vi "Temperature Warnings_EX.vi"() -> ()   [LabVIEW 2021]
doc: "This VI is used to determine the string to output to the weather station based on the current temperature and limit settings.\n\nInputs: Current Temperature (DBL), Minimum Temperature (DBL), and Maximum Temperature (DBL).\nOutputs: Warning Text (string) and Warning? (Boolean)."
uses:
  WeatherData.ctl
panel:
  out "Weather Out":T1={"Current Temperature"=0.0, "Max Temperature"=0.0, "Min Temperature"=0.0, "Warning?"=FALSE, "Warning Text"="No Warning"}
  in  "Weather In":T1={"Current Temperature"=0.0, "Max Temperature"=0.0, "Min Temperature"=0.0, "Warning?"=FALSE, "Warning Text"="No Warning"}
  out "Error Out":errorcluster
  in  "Error In":errorcluster
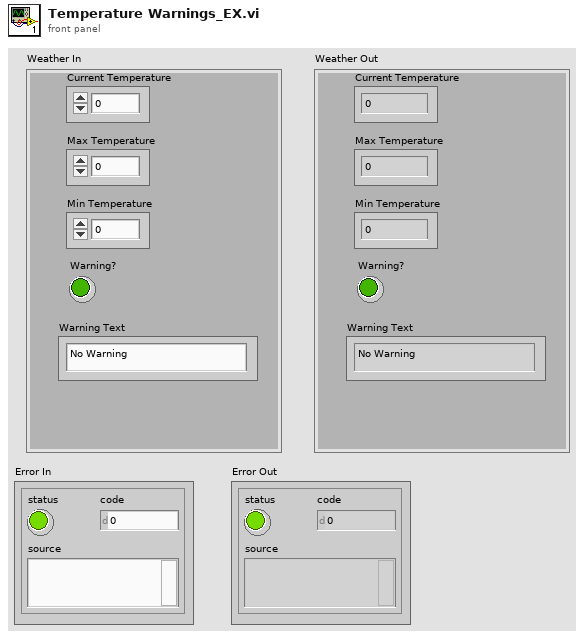
[diagram p1: front panel]
types:
  T1 = typedef "WeatherData.ctl" = cluster{"Current Temperature":dbl, "Max Temperature":dbl, "Min Temperature":dbl, "Warning?":bool, "Warning Text":string}
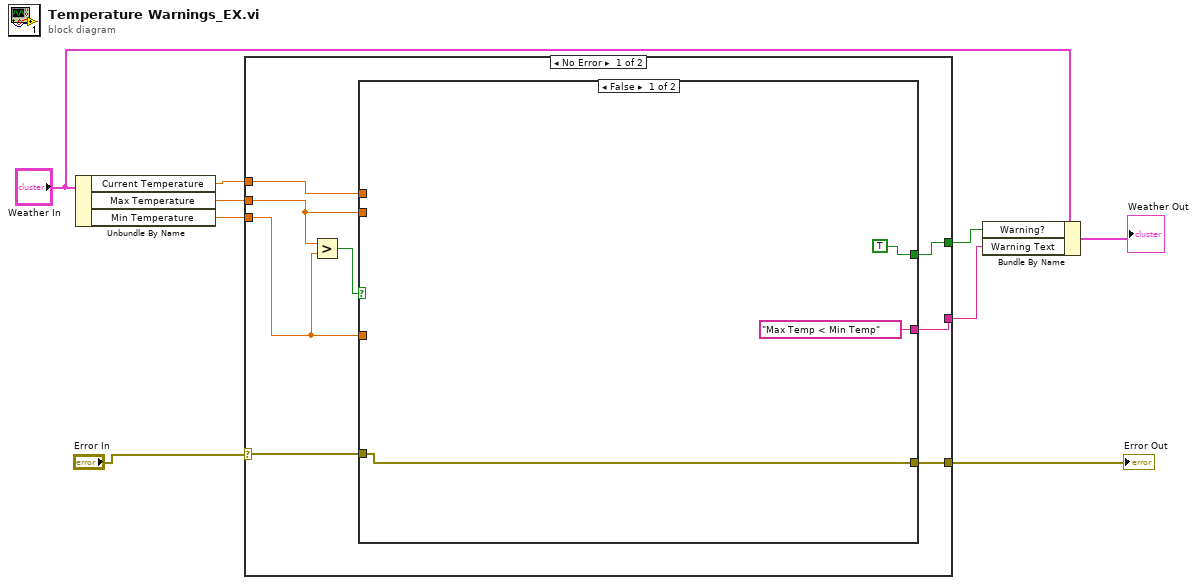
[diagram p0: block diagram]
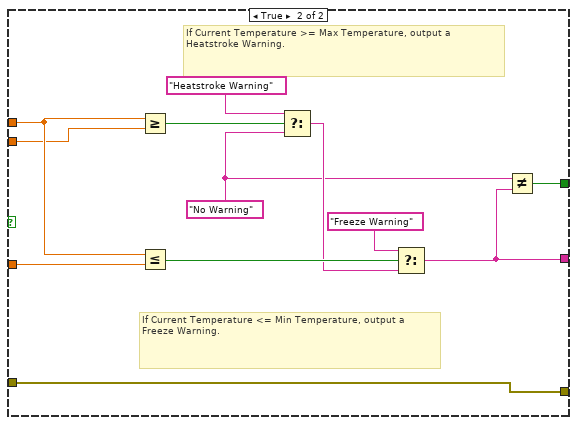
[diagram p2: hidden frame]
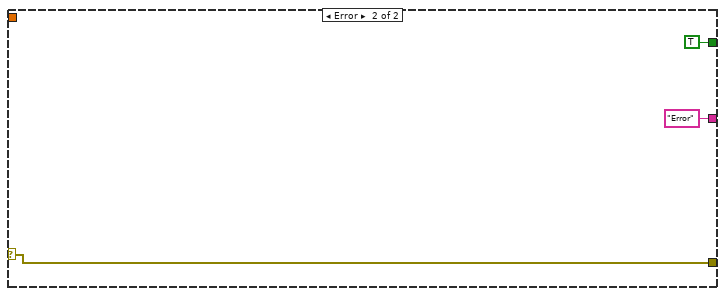
[diagram p3: hidden frame]
diagram:
  n1 = Unbundle By Name("Weather In") -> ("Current Temperature"=w9:dbl, "Max Temperature"=w8:dbl, "Min Temperature"=w7:dbl)
  n2 = case shown="No Error" "Error In" {
    selector: "Error In" -> [w10 w33]
    tunnel: w9 -> [w17 _]
    tunnel: w8 -> [w14 _]
    tunnel: w7 -> [w13 _]
    tunnel: [w16 TRUE] -> w5
    tunnel: [w15 "Error" ("f")] -> w4
    tunnel: [w11 w33] -> w1
    frame No Error {
      n3 = Greater?(x=w14, y=w13) -> (0:w12:bool)
      n4 = case shown="False" w12 {
        tunnel: w17 -> [_ w26]
        tunnel: w14 -> [_ w25]
        tunnel: w13 -> [_ w24]
        tunnel: [TRUE w23] -> w16
        tunnel: ["Max Temp < Min Temp" ("f") w22] -> w15
        tunnel: [w18 w21] -> w11
        tunnel: w10 -> [w18 w21]
        frame False {
        }
        frame True {
          w27 = "No Warning" ("f")
          # "If Current Temperature >= Max Temperature, output a Heatstroke Warning."
          # "If Current Temperature <= Min Temperature, output a Freeze Warning."
          n5 = Greater Or Equal?(x=w26, y=w25) -> (x >= y?=w32:bool)
          n6 = Less Or Equal?(x=w26, y=w24) -> (x <= y?=w29:bool)
          n7 = Select(t="Heatstroke Warning", s=w32, f=w27) -> (s? t:f=w28:string)
          n8 = Select(t="Freeze Warning", s=w29, f=w28) -> (s? t:f=w22:string)
          n9 = Not Equal?(x=w27, y=w22) -> (x != y?=w23:bool)
        }
      }
    }
    frame Error {
    }
  }
  "Error Out" <- w1
  n10 = Bundle By Name(cluster="Weather In", "Warning?"=w5, "Warning Text"=w4) -> (→"Weather Out":T1)
